vi "Assemble Subarray.vi"(8 "error in":errorcluster, 10 "Rx record":T1 {"type" format="%04x"; "activity" format="%04x"; "error" format="%04x"; "cwd1" format="%04x"; "cwd2" format="%04x"; "swd1" format="%04x"; "swd2" format="%04x"; "data" format="%04x"}, 11 "message":T2) -> (0 "error out":errorcluster, 2 "subarray":dbl[](array[numeric]), 3 "value indexes":i32[](array[numeric]))   [LabVIEW 2020, in "Ballard MIL-STD-1553 Engine.lvlib" / "Implementation.lvlib" / "Rx Execution Unit.lvclass"]
uses:
  Rx Execution Unit.lvclass
  Message Map Value.ctl
  Shared/Message Definition.ctl
  Shared/Message Type.ctl
  Shared/Terminal Endpoint.ctl
  Shared/Address.ctl
  Shared/Parameter Definition.ctl
  <instrlib>/BTICardLib/Public/Controls/1553 Record.ctl
  <instrlib>/BTICardLib/BTICardLV.lvlib
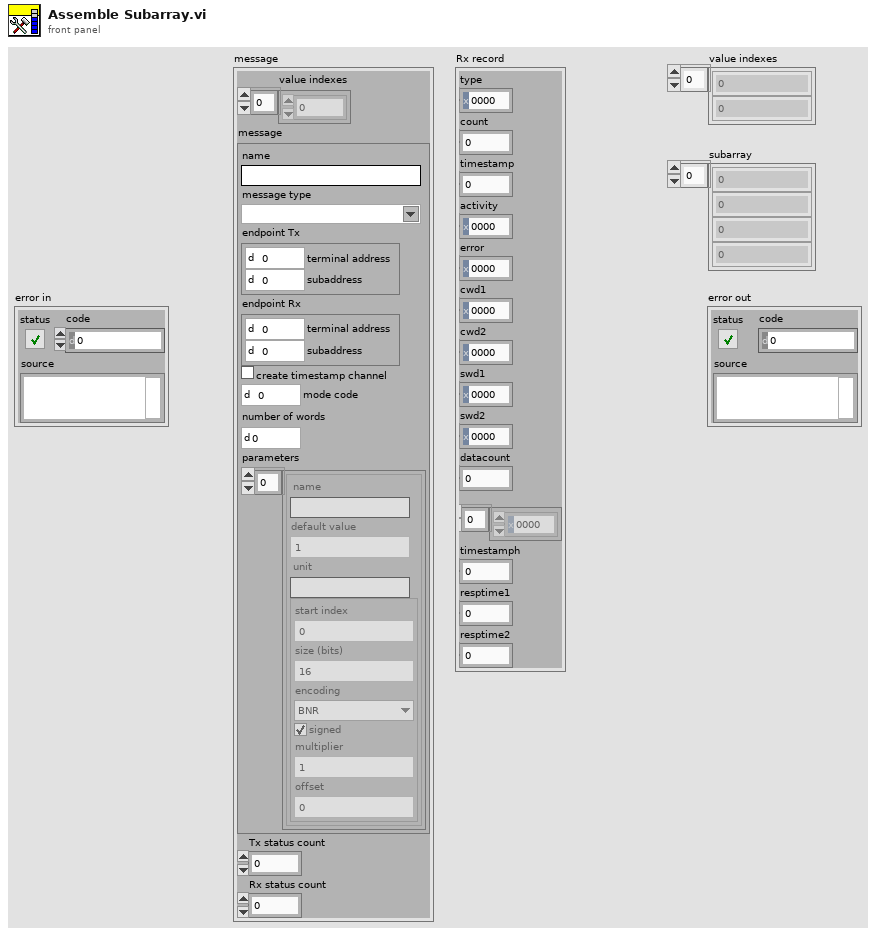
[diagram p1: front panel]
types:
  T1 = typedef "BTICardLV.lvlib/1553 Record.ctl" = cluster{"type":u16, "count":u16, "timestamp":u32, "activity":u16, "error":u16, "cwd1":u16, "cwd2":u16, "swd1":u16, "swd2":u16, "datacount":u16, "data":u16[], "timestamph":u32, "resptime1":u16, "resptime2":u16}
  T2 = typedef "Ballard MIL-STD-1553 Engine.lvlib/Implementation.lvlib/Rx Execution Unit.lvclass/Message Map Value.ctl" = cluster{"value indexes":i32[], "message":T3, "Tx status count":i32, "Rx status count":i32}
  T3 = typedef "Message Definition.ctl" = cluster{"name":string, "message type":T4, "endpoint Tx":T5, "endpoint Rx":T5, "create timestamp channel":bool, "mode code":u16, "number of words":u16, "parameters":cluster{"name":string, "default value":dbl, "unit":string, "parameter definition":T7}[]}
  T4 = typedef "Message Type.ctl" = string
  T5 = typedef "Terminal Endpoint.ctl" = cluster{"terminal address":T6, "subaddress":T6}
  T6 = typedef "Address.ctl" = u16
  T7 = typedef "Parameter Definition.ctl" = cluster{"start index":i32, "size (bits)":i32, "encoding":enum16{"BNR", "BCD", "Discrete"}, "signed":bool, "multiplier":dbl, "offset":dbl}
  T8 = cluster{"name":string, "default value":dbl, "unit":string, "parameter definition":T7}[]
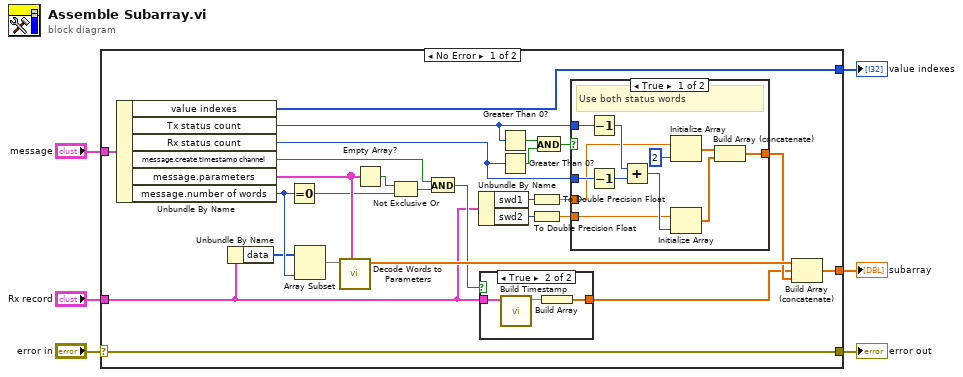
[diagram p0: block diagram]
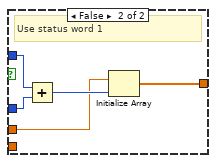
[diagram p3: hidden frame]
diagram:
  n1 = case shown="No Error" "error in" {
    selector: "error in" -> [w17 w52]
    tunnel: "message" -> [w31 _]
    tunnel: [w30 _] -> w5
    tunnel: "Rx record" -> [w7 _]
    tunnel: [w19 _] -> w3
    tunnel: [w17 w52] -> w1
    frame No Error {
      n2 = Unbundle By Name(w31) -> ("value indexes"=w19:i32[], "Tx status count"=w20:i32, "Rx status count"=w21:i32, "message.create timestamp channel"=w10:bool, "message.parameters"=w15:T8, "message.number of words"=w14:u16)
      n3 = Unbundle By Name(w7) -> ("data"=w8:u16[])
      n4 = Equal To 0?(x=w14) -> (x = 0?=w12:bool)
      n5 = Array Subset(array=w8, length=w14) -> (w16:u16[])  [unwired: 1 in]
      n6 = call "Decode Words to Parameters.vi"("parameters"=w15, "data words"=w16) -> ("Values"=w32:dbl[])  [unwired: 9 in]
      n7 = Empty Array?(array=w15) -> (empty?=w13:bool)
      n8 = Not Exclusive Or(1:w12, 2:w13) -> (0:w11:bool)
      n9 = And(x=w10, y=w11) -> (x .and. y?=w9:bool)
      n10 = Unbundle By Name(w7) -> ("swd1"=w23:u16, "swd2"=w22:u16)
      n11 = case shown="True" w9 {
        tunnel: [_ w33] -> w18
        tunnel: w7 -> [_ w35]
        frame False {
        }
        frame True {
          n12 = call "Build Timestamp.vi"("record"=w35) -> ("timestamp"=w34:dbl)  [unwired: 10 in]
          n13 = Build Array(w34) -> (w33:dbl[])
        }
      }
      n14 = Greater Than 0?(x=w20) -> (x > 0?=w25:bool)
      n15 = Greater Than 0?(x=w21) -> (x > 0?=w24:bool)
      n16 = To Double Precision Float(number=w23) -> (double precision float=w27:dbl)
      n17 = To Double Precision Float(number=w22) -> (double precision float=w28:dbl)
      n18 = And(x=w25, y=w24) -> (x .and. y?=w26:bool)
      n19 = case shown="True" w26 {
        tunnel: w21 -> [w43 w50]
        tunnel: [w46 w49] -> w29
        tunnel: w20 -> [w38 w48]
        tunnel: w27 -> [w37 w47]
        tunnel: w28 -> [w36 _]
        frame True {
          # "Use both status words"
          n20 = Decrement(x=w38) -> (x-1=w41:i32)
          n21 = Decrement(x=w43) -> (x-1=w42:i32)
          n22 = Add(x=w41, y=w42) -> (x+y=w39:i32)
          n23 = Initialize Array(w37, 2 ("dimension size")) -> (w45:dbl[])
          n24 = Initialize Array(w36, w39) -> (w40:dbl[])
          n25 = Build Array (concatenate)(w45, w40) -> (w46:dbl[])
        }
        frame False {
          # "Use status word 1"
          n26 = Add(x=w48, y=w50) -> (x+y=w51:i32)
          n27 = Initialize Array(w47, w51) -> (w49:dbl[])
        }
      }
      n28 = Build Array (concatenate)(w32, w18, w29) -> (w30:dbl[])
    }
    frame Error {
    }
  }
  "subarray" <- w5
  "value indexes" <- w3
  "error out" <- w1
